vi "repPreparePenaltyEnemyPlayVSS.vi"(8 "error in (no error)":errorcluster, 9 "Game in 2":refnum<class "Game.lvclass">, 10 "RobotPlacement":T1(array[cluster]), 11 "PreparePenaltyEnemyPlayVSS in":refnum<class "PreparePenaltyEnemyPlayVSS.lvclass">) -> (0 "error out":errorcluster, 2 "RobotPlacement 2":T1(array[cluster]), 3 "PreparePenaltyEnemyPlayVSS out":refnum<class "PreparePenaltyEnemyPlayVSS.lvclass">)   [LabVIEW 2020, in "PreparePenaltyEnemyPlayVSS.lvclass"]
uses:
  PreparePenaltyEnemyPlayVSS.lvclass
  Game_class/Game.lvclass
  Game_class/Game.lvclass/Game.ctl
  Game_class/Read FieldRef.vi
  Field_class/Field.lvclass
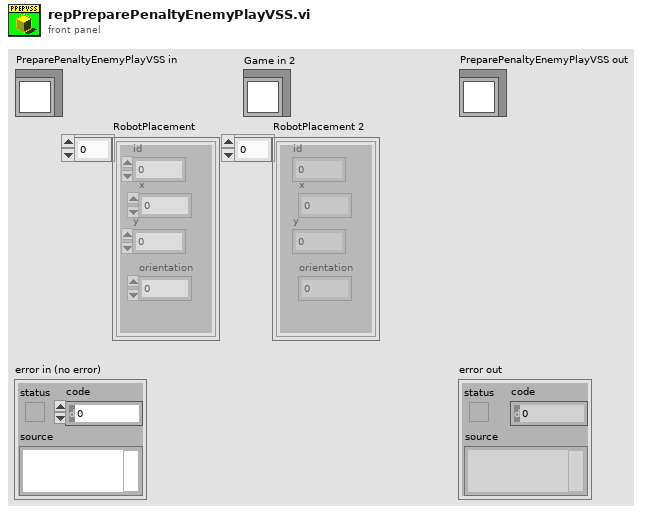
[diagram p1: front panel]
types:
  T1 = cluster{"id":i32, "x":dbl, "y":dbl, "orientation":dbl}[]
  T2 = cluster{"id":i32, "x":dbl, "y":dbl, "orientation":dbl}
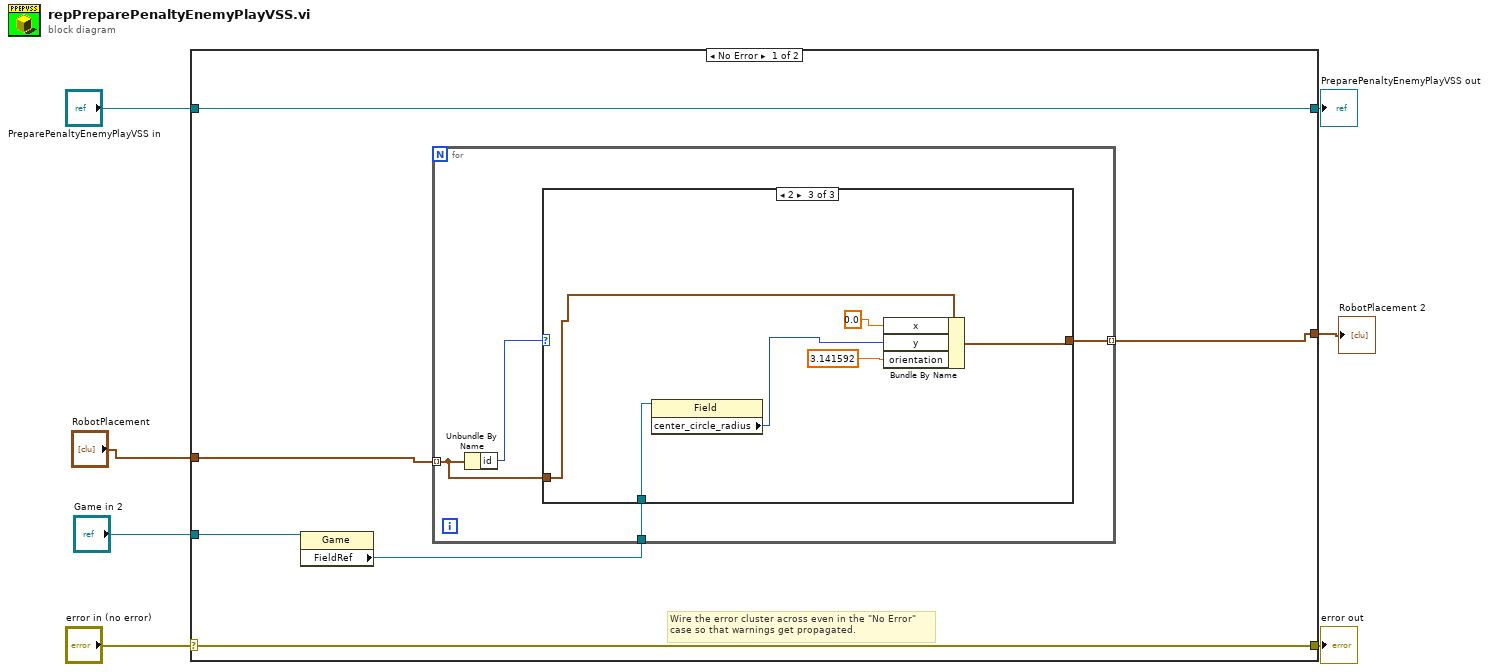
[diagram p0: block diagram]
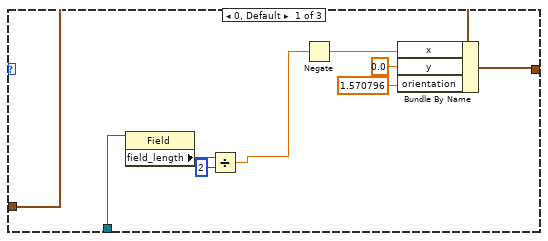
[diagram p2: hidden frame]
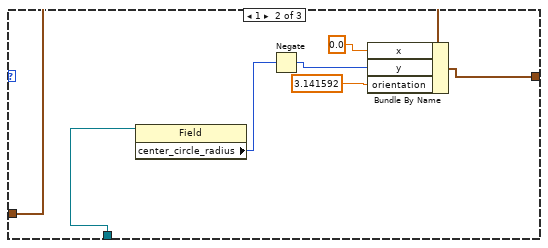
[diagram p3: hidden frame]
diagram:
  n1 = case shown="No Error" "error in (no error)" {
    selector: "error in (no error)" -> [w12 w41]
    tunnel: [w12 w41] -> w6
    tunnel: [w13 w40] -> w4
    tunnel: "PreparePenaltyEnemyPlayVSS in" -> [w13 w40]
    tunnel: [w10 _] -> w3
    tunnel: "RobotPlacement" -> [w9 _]
    tunnel: "Game in 2" -> [w8 _]
    frame No Error {
      # "Wire the error cluster across even in the \"No Error\"\ncase so that warnings get propagated."
      n2 = property class="Game"(reference=w8) -> ("FieldRef"=w11:refnum<class "Field.lvclass">)  [unwired: 1 in, 2 out]
      n3 = for {
        tunnel: w9 -> [w16] mode=indexing
        tunnel: [w15] -> w10 mode=indexing
        tunnel: w11 -> [w14]
        n4 = Unbundle By Name(w16) -> ("id"=w17:i32)
        n5 = case shown="2" w17 {
          tunnel: w16 -> [w26 w33 w37]
          tunnel: [w25 w32 w36] -> w15
          tunnel: w14 -> [w24 w31 w34]
          frame 0, Default {
            n6 = property class="Field"(reference=w24) -> ("field_length"=w23:i32)  [unwired: 1 in, 2 out]
            n7 = Divide(x=w23, y=2) -> (x/y=w19:dbl)
            n8 = Negate(x=w19) -> (-x=w18:dbl)
            n9 = Bundle By Name(cluster=w26, "x"=w18, "y"=0.0, "orientation"=1.570796) -> (w25:T2)
          }
          frame 1 {
            n10 = property class="Field"(reference=w31) -> ("center_circle_radius"=w28:i32)  [unwired: 1 in, 2 out]
            n11 = Negate(x=w28) -> (-x=w27:i32)
            n12 = Bundle By Name(cluster=w33, "x"=0.0, "y"=w27, "orientation"=3.141592 ("x")) -> (w32:T2)
          }
          frame 2 {
            n13 = property class="Field"(reference=w34) -> ("center_circle_radius"=w35:i32)  [unwired: 1 in, 2 out]
            n14 = Bundle By Name(cluster=w37, "x"=0.0, "y"=w35, "orientation"=3.141592 ("x")) -> (w36:T2)
          }
        }
      }
    }
    frame Error {
    }
  }
  "error out" <- w6
  "PreparePenaltyEnemyPlayVSS out" <- w4
  "RobotPlacement 2" <- w3
